vi "CCMD DSP402.vi"(4 "error in (no error)":errorcluster, 6 "Mask":T1[](array[typedef]) items=["---", "OFF", "ON"], 7 "DSP402 in":refnum<class "DSP402.lvclass">) -> (0 "error out":errorcluster, 3 "DSP402 out":refnum<class "DSP402.lvclass">)   [LabVIEW 2024, in "canopen.lvlib" / "DSP402.lvclass"]
uses:
  DSP402.lvclass
  types/threestateFlag.ctl
  DSP402.lvclass/DSP402.ctl
  canopen.lvlib
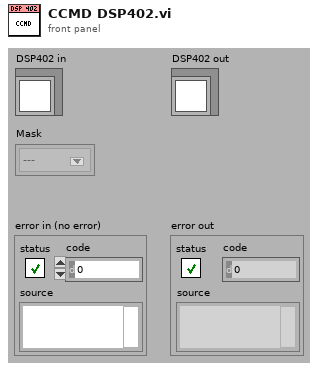
[diagram p1: front panel]
types:
  T1 = typedef "canopen.lvlib/threestateFlag.ctl" = i8
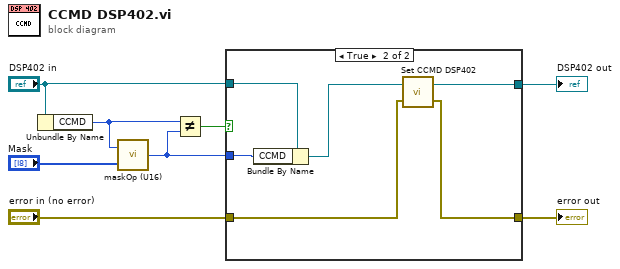
[diagram p0: block diagram]
diagram:
  n1 = Unbundle By Name("DSP402 in") -> ("CCMD"=w2:u16)
  n2 = call "maskOp (U16).vi"("Mask"="Mask", "Original"=w2) -> ("Result"=w3:u16)
  n3 = Not Equal?(x=w2, y=w3) -> (x != y?=w5:bool)
  n4 = case shown="True" w5 {
    tunnel: "error in (no error)" -> [w10 w11]
    tunnel: [w10 w12] -> w7
    tunnel: w3 -> [_ w16]
    tunnel: "DSP402 in" -> [w9 w15]
    tunnel: [w9 w13] -> w4
    frame False {
    }
    frame True {
      n5 = Bundle By Name(cluster=w15, "CCMD"=w16) -> (w14:refnum<class "DSP402.lvclass">)
      n6 = call "Set CCMD DSP402.vi"("error in (no error)"=w11, "DSP402 in"=w14) -> ("error out"=w12:errorcluster, "DSP402 out"=w13:refnum<class "DSP402.lvclass">)
    }
  }
  "error out" <- w7
  "DSP402 out" <- w4
